vi "InitArm.vi"   [LabVIEW 2020]
uses:
  <vilib>/Rock Robotics/WPI/ThirdParty/Phoenix-LabVIEW/Motor Controller/Controls/CTRE_Phoenix_MotorControl_TalonFXInvertType.ctl
  <vilib>/Rock Robotics/WPI/ThirdParty/Phoenix-LabVIEW/Motor Controller/Controls/CTRE_Phoenix_MotorControl_NeutralMode.ctl
  <vilib>/Rock Robotics/WPI/ThirdParty/Phoenix-LabVIEW/Motor Controller/Controls/CTRE_Phoenix_MotorControl_FeedbackDevice_TalonFX.ctl
  <vilib>/Rock Robotics/WPI/ThirdParty/Phoenix-LabVIEW/Motor Controller/Controls/CTRE_Phoenix_MotorControl_SupplyCurrentLimitConfiguration.ctl
  <vilib>/Rock Robotics/WPI/ThirdParty/Phoenix-LabVIEW/Motor Controller/Controls/CTRE_Phoenix_MotorControl_StatusFrameEnhanced.ctl
  <vilib>/robotics/Kinematics/DH Kinematic Parameters.ctl
  <vilib>/robotics/Kinematics/Link/Joint Type.ctl
  <vilib>/robotics/Kinematics/DH Dynamic Parameters.ctl
  <vilib>/Analysis/Matrix/Datatypes/RealMatrix.ctl
  <vilib>/robotics/Kinematics/RotateX.vi
  <vilib>/robotics/Kinematics/RotateY.vi
  <vilib>/robotics/Kinematics/RotateZ.vi
  <vilib>/Analysis/baseanly.llb/A x B.vi
  <vilib>/Analysis/baseanly.llb/Real A x B.vi
  GlobalArm.vi
  <vilib>/robotics/Kinematics/Analytical/Initialize Generic Serial Arm.vi
  <vilib>/robotics/Kinematics/Robot/NI_Robotics_Serial Robot Arm.lvclass
  <vilib>/robotics/Kinematics/Link/NI_Robotics_Link.lvclass
  <vilib>/robotics/Kinematics/NI_Kinematics.lvlib
  <vilib>/Analysis/Matrix/NI_Matrix.lvlib
  <vilib>/robotics/Kinematics/Analytical/NI_Robotics_AnalyticKinematics.lvlib
types:
  T1 = typedef "CTRE_Phoenix_MotorControl_SupplyCurrentLimitConfiguration.ctl" = cluster{"Enable?":bool, "Current Limit":dbl, "Threshold Current":dbl, "Threshold Time":dbl}
  T2 = typedef "CTRE_Phoenix_MotorControl_NeutralMode.ctl" = enum8{"EEPROMSetting", "Override to Coast", "Override to Brake"}
  T3 = typedef "CTRE_Phoenix_MotorControl_TalonFXInvertType.ctl" = enum16{"Counter-Clockwise", "Clockwise"}
  T4 = typedef "DH Kinematic Parameters.ctl" = cluster{"twist angle":dbl, "length":dbl, "rotation angle":dbl, "offset distance":dbl, "joint type":T5, "joint coordinate offset":dbl}
  T5 = typedef "NI_Robotics_Link.lvclass/Joint Type.ctl" = enum16{"Revolute", "Prismatic"}
  T6 = typedef "CTRE_Phoenix_MotorControl_StatusFrameEnhanced.ctl" = u16
  T7 = typedef "CTRE_Phoenix_MotorControl_FeedbackDevice_TalonFX.ctl" = i8
  T8 = typedef "WPI_MotorControlDeviceRef.ctl" = cluster{"DeviceStatus":errorcluster, "Type":T9, "PWM":cluster{"PWM Channel":T10, "DeadBand":T11}, "CAN":cluster{"Device Number":u8, "SetOutput VI Ref":variant, "GetOutput VI Ref":variant, "Enable VI Ref":variant, "Disable VI Ref":variant, "Data":variant}, "Invert":bool, "DIO PWM":cluster{"PWM \"Enable\" Channel":T10, "DIOChannel":T12, "PWM Rate":dbl}}
  T9 = typedef "WPI_MotorControlType.ctl" = enum16{"PWM", "CAN", "DIO PWM"}
  T10 = typedef "FPGA_DIOPWMChannel.ctl" = enum8{"PWM 0", "PWM 1", "PWM 2", "PWM 3", "PWM 4", "PWM 5", "PWM 6", "PWM 7", "PWM 8", "PWM 9", "PWM MXP 0", "PWM MXP 1", "PWM MXP 2", "PWM MXP 3", "PWM MXP 4", "PWM MXP 5", "PWM MXP 6", "PWM MXP 7", "PWM MXP 8", "PWM MXP 9", "Invalid"}
  T11 = typedef "WPI_PWMDeadband.ctl" = cluster{"Name":string, "maxPositivePwm":i32, "minPositivePwm":i32, "centerPwm":i32, "maxNegativePwm":i32, "minNegativePwm":i32, "angularRange":u16}
  T12 = typedef "FPGA_DIOChannel.ctl" = enum8{"DIO 0", "DIO 1", "DIO 2", "DIO 3", "DIO 4", "DIO 5", "DIO 6", "DIO 7", "DIO 8", "DIO 9", "DIO MXP 0", "DIO MXP 1", "DIO MXP 2", "DIO MXP 3", "DIO MXP 4", "DIO MXP 5", "DIO MXP 6", "DIO MXP 7", "DIO MXP 8", "DIO MXP 9", "DIO MXP 10", "DIO MXP 11", "DIO MXP 12", "DIO MXP 13", "DIO MXP 14", "DIO MXP 15", "SPI Port CS1", "SPI Port CS2", "SPI Port CS3", "SPI Port MISO", "SPI Port MOSI", "Invalid"}
  T13 = typedef "DH Dynamic Parameters.ctl" = cluster{"mass":dbl, "gear ratio":dbl, "motor inertia":dbl, "center of gravity":dbl[], "viscous friction":dbl, "positive coulomb friction":dbl, "negative coulomb friction":dbl, "inertia matrix":T14}
  T14 = typedef "NI_Matrix.lvlib/RealMatrix.ctl" = dbl[][]
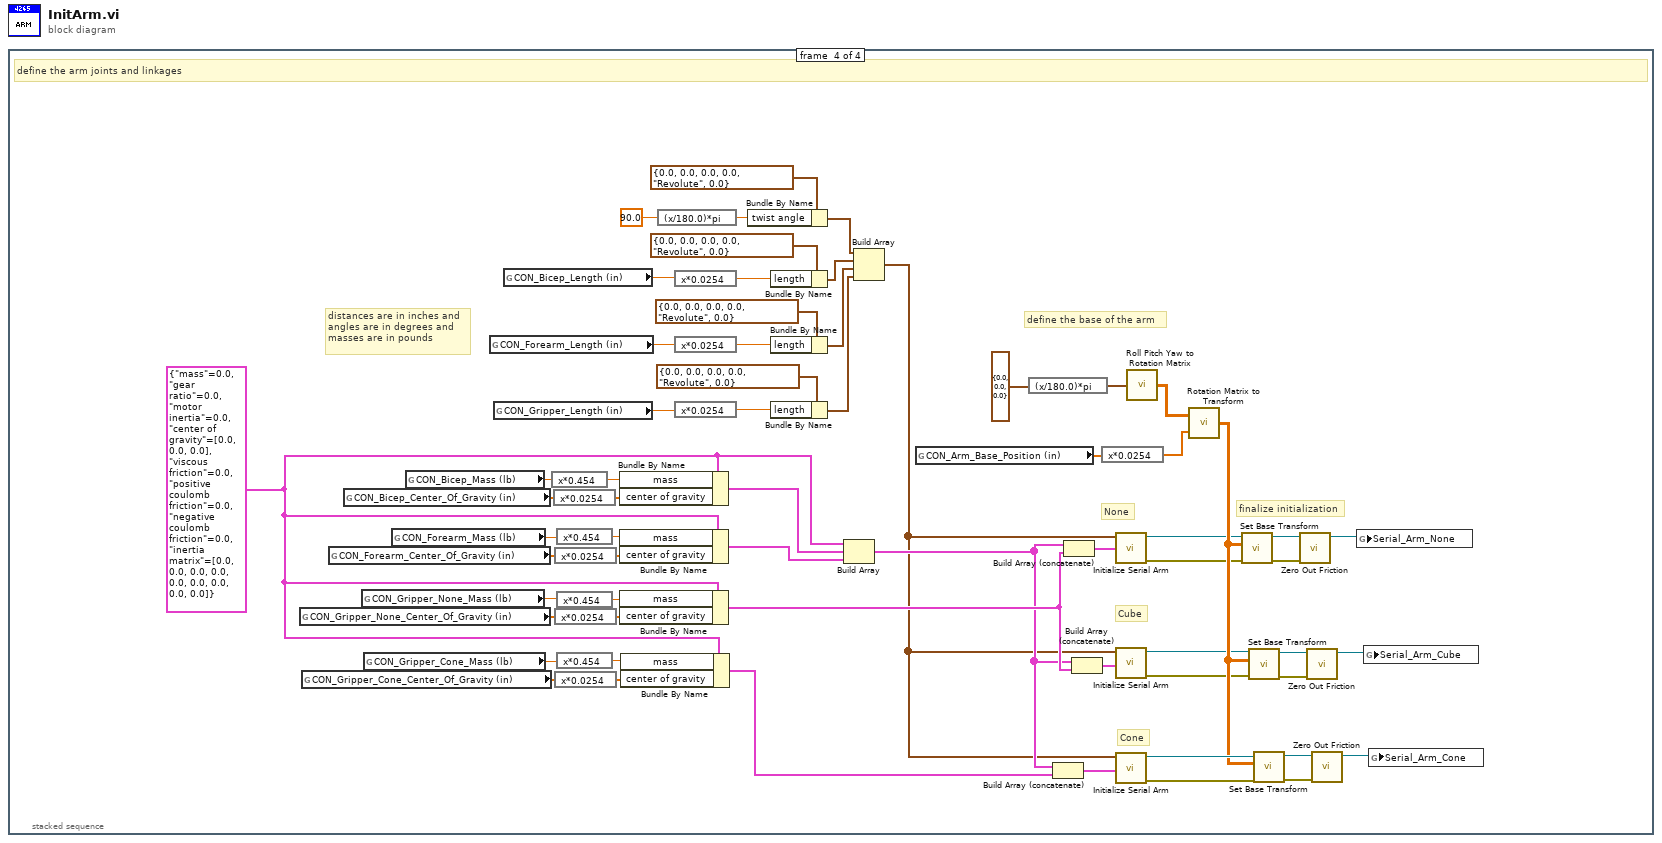
[diagram p0: block diagram]
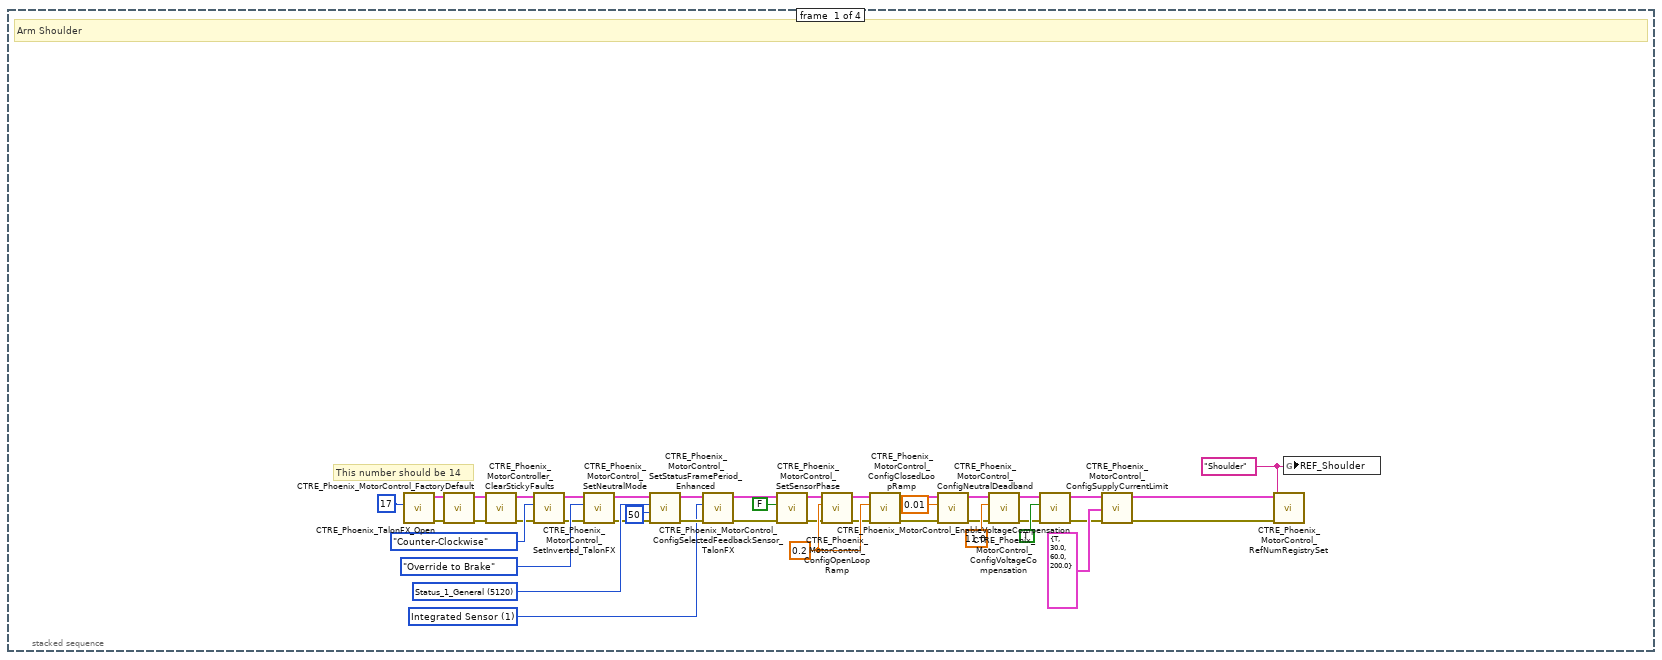
[diagram p2: hidden frame]
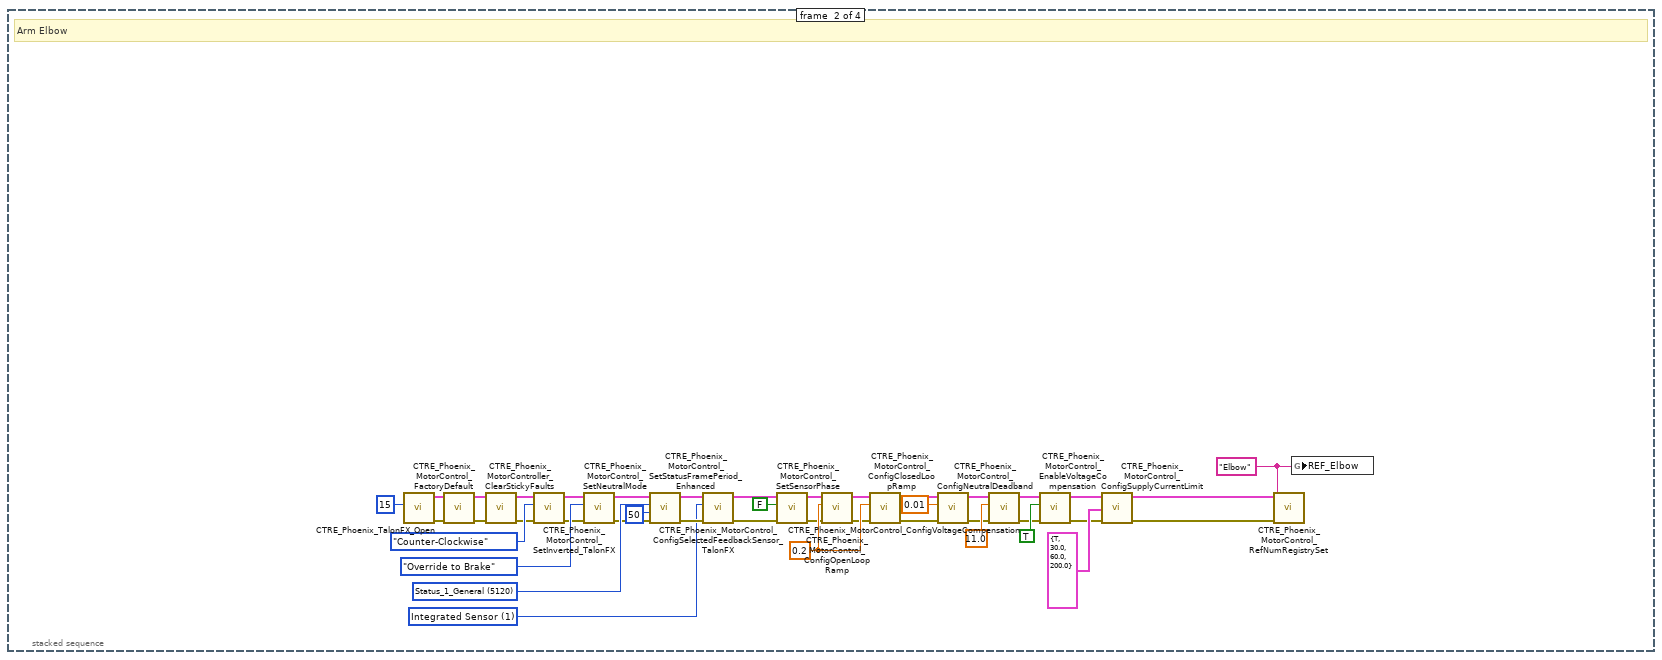
[diagram p3: hidden frame]
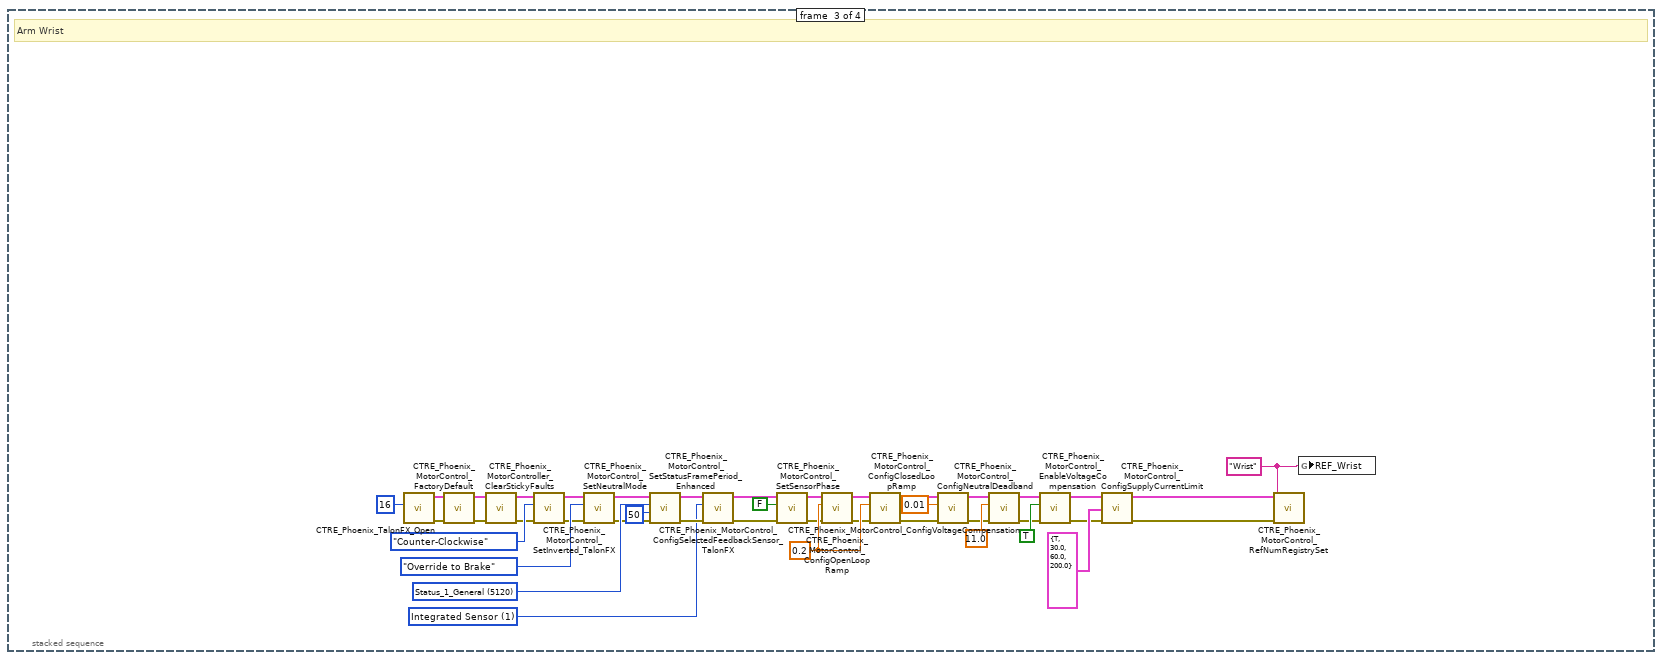
[diagram p4: hidden frame]
diagram:
  n1 = stacked-sequence {
    frame #0 {
      w23 = T6 5120 items=["Status_1_General"=5120, "Status_2_Feedback0"=5184, "Status_3_Quadrature"=5248, "Status_4_AinTempVbat"=5312, "Status_6_Misc"=5440, "Status_7_CommStatus"=5504, "Status_8_PulseWidth"=5568, "Status_9_MotProfBuffer"=5632, "Status_10_MotionMagic"=5696, "Status_11_UartGadgeteer"=5760, "Status_12_Feedback1"=5824, "Status_13_Base_PIDF0"=5888, "Status_14_Turn_PIDF1"=5952, "Status_15_FirmwareApiStatus"=6016, "Status_Brushless_Current"=4672] ("Status Frame")
      w24 = "Shoulder" ("refnum name")
      w28 = 0.2 ("secondsFromNeutralToFull")
      w1 = T7 1 items=["Integrated Sensor"=1, "Sensor Sum (S0 + S1)"=9, "Sensor Difference (D0 - D1)"=10, "Remote Source 0"=11, "Remote Source 1"=12, "None"=14, "Software Emulated"=15] ("Talon FX Feedback Device")
      # "This number should be 14"
      # "Arm Shoulder"
      n2 = call <vilib>:"CTRE_Phoenix_TalonFX_Open.vi"("Device Number"=u8 17) -> ("error out"=w16:errorcluster, "PhoenixMotorControlDevRef"=w33:T8)  [unwired: 9 in]
      n3 = call <vilib>:"CTRE_Phoenix_MotorControl_FactoryDefault.vi"("error in"=w16, "PhoenixMotorControlDevRef"=w33) -> ("error out"=w17:errorcluster, "PhoenixMotorControlDevRef"=w34:T8)  [unwired: 8 in]
      n4 = call <vilib>:"CTRE_Phoenix_MotorController_ClearStickyFaults.vi"("error in"=w17, "PhoenixMotorControlDevRef"=w34) -> ("error out"=w18:errorcluster, "PhoenixMotorControlDevRef"=w35:T8)  [unwired: 8 in]
      n5 = call <vilib>:"CTRE_Phoenix_MotorControl_SetInverted_TalonFX.vi"("error in (no error)"=w18, "Invert Type"=CTRE_Phoenix_MotorControl_TalonFXInvertType."Counter-Clockwise", "PhoenixMotorControlDevRef"=w35) -> ("error out"=w19:errorcluster, "PhoenixMotorControlDevRef"=w36:T8)  [unwired: 7 in]
      n6 = call <vilib>:"CTRE_Phoenix_MotorControl_SetNeutralMode.vi"("error in (no error)"=w19, "Motor Control Neutral Mode"=CTRE_Phoenix_MotorControl_NeutralMode."Override to Brake", "PhoenixMotorControlDevRef"=w36) -> ("error out"=w20:errorcluster, "PhoenixMotorControlDevRef"=w41:T8)  [unwired: 7 in]
      n7 = call <vilib>:"CTRE_Phoenix_MotorControl_SetStatusFramePeriod_Enhanced.vi"("error in (no error)"=w20, "periodMs"=50, "Status Frame"=w23, "PhoenixMotorControlDevRef"=w41) -> ("error out"=w21:errorcluster, "PhoenixMotorControlDevRef"=w22:T8)  [unwired: 6 in]
      n8 = call <vilib>:"CTRE_Phoenix_MotorControl_ConfigSelectedFeedbackSensor_TalonFX.vi"("error in (no error)"=w21, "Talon FX Feedback Device"=w1, "PhoenixMotorControlDevRef"=w22) -> ("error out"=w9:errorcluster, "PhoenixMotorControlDevRef"=w11:T8)  [unwired: 7 in]
      n9 = call <vilib>:"CTRE_Phoenix_MotorControl_SetSensorPhase.vi"("error in (no error)"=w9, "PhaseSensor"=FALSE, "PhoenixMotorControlDevRef"=w11) -> ("error out"=w8:errorcluster, "PhoenixMotorControlDevRef"=w10:T8)  [unwired: 7 in]
      n10 = call <vilib>:"CTRE_Phoenix_MotorControl_ConfigOpenLoopRamp.vi"("error in (no error)"=w8, "secondsFromNeutralToFull"=w28, "PhoenixMotorControlDevRef"=w10) -> ("error out"=w15:errorcluster, "PhoenixMotorControlDevRef"=w37:T8)  [unwired: 7 in]
      n11 = call <vilib>:"CTRE_Phoenix_MotorControl_ConfigClosedLoopRamp.vi"("error in (no error)"=w15, "secondsFromNeutralToFull"=w28, "PhoenixMotorControlDevRef"=w37) -> ("error out"=w5:errorcluster, "PhoenixMotorControlDevRef"=w6:T8)  [unwired: 7 in]
      n12 = call <vilib>:"CTRE_Phoenix_MotorControl_ConfigNeutralDeadband.vi"("error in (no error)"=w5, "Percent Deadband"=0.01, "PhoenixMotorControlDevRef"=w6) -> ("error out"=w4:errorcluster, "PhoenixMotorControlDevRef"=w3:T8)  [unwired: 7 in]
      n13 = call <vilib>:"CTRE_Phoenix_MotorControl_ConfigVoltageCompensation.vi"("error in (no error)"=w4, "Saturation Voltage"=11.0, "PhoenixMotorControlDevRef"=w3) -> ("error out"=w14:errorcluster, "PhoenixMotorControlDevRef"=w38:T8)  [unwired: 7 in]
      n14 = call <vilib>:"CTRE_Phoenix_MotorControl_EnableVoltageCompensation.vi"("error in (no error)"=w14, "Enable Voltage Compensation?"=TRUE, "PhoenixMotorControlDevRef"=w38) -> ("error out"=w13:errorcluster, "PhoenixMotorControlDevRef"=w39:T8)  [unwired: 7 in]
      n15 = call <vilib>:"CTRE_Phoenix_MotorControl_ConfigSupplyCurrentLimit.vi"("error in (no error)"=w13, "Supply Current Limit Configuration"=T1 {"Enable?"=TRUE, "Current Limit"=30.0, "Threshold Current"=60.0, "Threshold Time"=200.0}, "PhoenixMotorControlDevRef"=w39) -> ("error out"=w12:errorcluster, "PhoenixMotorControlDevRef"=w40:T8)  [unwired: 7 in]
      n16 = call <vilib>:"CTRE_Phoenix_MotorControl_RefNumRegistrySet.vi"("error in (no error)"=w12, "refnum name"=w24, "PhoenixMotorControlDevRef"=w40) -> ()  [unwired: 7 in, 2 out]
      n17 = global write "GlobalArm.vi" "REF_Shoulder"(w24) -> ()
    }
    frame #1 {
      w64 = T6 5120 items=["Status_1_General"=5120, "Status_2_Feedback0"=5184, "Status_3_Quadrature"=5248, "Status_4_AinTempVbat"=5312, "Status_6_Misc"=5440, "Status_7_CommStatus"=5504, "Status_8_PulseWidth"=5568, "Status_9_MotProfBuffer"=5632, "Status_10_MotionMagic"=5696, "Status_11_UartGadgeteer"=5760, "Status_12_Feedback1"=5824, "Status_13_Base_PIDF0"=5888, "Status_14_Turn_PIDF1"=5952, "Status_15_FirmwareApiStatus"=6016, "Status_Brushless_Current"=4672] ("Status Frame")
      w65 = "Elbow" ("refnum name")
      w69 = 0.2 ("secondsFromNeutralToFull")
      w42 = T7 1 items=["Integrated Sensor"=1, "Sensor Sum (S0 + S1)"=9, "Sensor Difference (D0 - D1)"=10, "Remote Source 0"=11, "Remote Source 1"=12, "None"=14, "Software Emulated"=15] ("Talon FX Feedback Device")
      # "Arm Elbow"
      n18 = call <vilib>:"CTRE_Phoenix_TalonFX_Open.vi"("Device Number"=u8 15) -> ("error out"=w57:errorcluster, "PhoenixMotorControlDevRef"=w74:T8)  [unwired: 9 in]
      n19 = call <vilib>:"CTRE_Phoenix_MotorControl_FactoryDefault.vi"("error in"=w57, "PhoenixMotorControlDevRef"=w74) -> ("error out"=w58:errorcluster, "PhoenixMotorControlDevRef"=w75:T8)  [unwired: 8 in]
      n20 = call <vilib>:"CTRE_Phoenix_MotorController_ClearStickyFaults.vi"("error in"=w58, "PhoenixMotorControlDevRef"=w75) -> ("error out"=w59:errorcluster, "PhoenixMotorControlDevRef"=w76:T8)  [unwired: 8 in]
      n21 = call <vilib>:"CTRE_Phoenix_MotorControl_SetInverted_TalonFX.vi"("error in (no error)"=w59, "Invert Type"=CTRE_Phoenix_MotorControl_TalonFXInvertType."Counter-Clockwise", "PhoenixMotorControlDevRef"=w76) -> ("error out"=w60:errorcluster, "PhoenixMotorControlDevRef"=w77:T8)  [unwired: 7 in]
      n22 = call <vilib>:"CTRE_Phoenix_MotorControl_SetNeutralMode.vi"("error in (no error)"=w60, "Motor Control Neutral Mode"=CTRE_Phoenix_MotorControl_NeutralMode."Override to Brake", "PhoenixMotorControlDevRef"=w77) -> ("error out"=w61:errorcluster, "PhoenixMotorControlDevRef"=w82:T8)  [unwired: 7 in]
      n23 = call <vilib>:"CTRE_Phoenix_MotorControl_SetStatusFramePeriod_Enhanced.vi"("error in (no error)"=w61, "periodMs"=50, "Status Frame"=w64, "PhoenixMotorControlDevRef"=w82) -> ("error out"=w62:errorcluster, "PhoenixMotorControlDevRef"=w63:T8)  [unwired: 6 in]
      n24 = call <vilib>:"CTRE_Phoenix_MotorControl_ConfigSelectedFeedbackSensor_TalonFX.vi"("error in (no error)"=w62, "Talon FX Feedback Device"=w42, "PhoenixMotorControlDevRef"=w63) -> ("error out"=w50:errorcluster, "PhoenixMotorControlDevRef"=w52:T8)  [unwired: 7 in]
      n25 = call <vilib>:"CTRE_Phoenix_MotorControl_SetSensorPhase.vi"("error in (no error)"=w50, "PhaseSensor"=FALSE, "PhoenixMotorControlDevRef"=w52) -> ("error out"=w49:errorcluster, "PhoenixMotorControlDevRef"=w51:T8)  [unwired: 7 in]
      n26 = call <vilib>:"CTRE_Phoenix_MotorControl_ConfigOpenLoopRamp.vi"("error in (no error)"=w49, "secondsFromNeutralToFull"=w69, "PhoenixMotorControlDevRef"=w51) -> ("error out"=w56:errorcluster, "PhoenixMotorControlDevRef"=w78:T8)  [unwired: 7 in]
      n27 = call <vilib>:"CTRE_Phoenix_MotorControl_ConfigClosedLoopRamp.vi"("error in (no error)"=w56, "secondsFromNeutralToFull"=w69, "PhoenixMotorControlDevRef"=w78) -> ("error out"=w46:errorcluster, "PhoenixMotorControlDevRef"=w47:T8)  [unwired: 7 in]
      n28 = call <vilib>:"CTRE_Phoenix_MotorControl_ConfigNeutralDeadband.vi"("error in (no error)"=w46, "Percent Deadband"=0.01, "PhoenixMotorControlDevRef"=w47) -> ("error out"=w45:errorcluster, "PhoenixMotorControlDevRef"=w44:T8)  [unwired: 7 in]
      n29 = call <vilib>:"CTRE_Phoenix_MotorControl_ConfigVoltageCompensation.vi"("error in (no error)"=w45, "Saturation Voltage"=11.0, "PhoenixMotorControlDevRef"=w44) -> ("error out"=w55:errorcluster, "PhoenixMotorControlDevRef"=w79:T8)  [unwired: 7 in]
      n30 = call <vilib>:"CTRE_Phoenix_MotorControl_EnableVoltageCompensation.vi"("error in (no error)"=w55, "Enable Voltage Compensation?"=TRUE, "PhoenixMotorControlDevRef"=w79) -> ("error out"=w54:errorcluster, "PhoenixMotorControlDevRef"=w80:T8)  [unwired: 7 in]
      n31 = call <vilib>:"CTRE_Phoenix_MotorControl_ConfigSupplyCurrentLimit.vi"("error in (no error)"=w54, "Supply Current Limit Configuration"=T1 {"Enable?"=TRUE, "Current Limit"=30.0, "Threshold Current"=60.0, "Threshold Time"=200.0}, "PhoenixMotorControlDevRef"=w80) -> ("error out"=w53:errorcluster, "PhoenixMotorControlDevRef"=w81:T8)  [unwired: 7 in]
      n32 = call <vilib>:"CTRE_Phoenix_MotorControl_RefNumRegistrySet.vi"("error in (no error)"=w53, "refnum name"=w65, "PhoenixMotorControlDevRef"=w81) -> ()  [unwired: 7 in, 2 out]
      n33 = global write "GlobalArm.vi" "REF_Elbow"(w65) -> ()
    }
    frame #2 {
      w106 = T6 5120 items=["Status_1_General"=5120, "Status_2_Feedback0"=5184, "Status_3_Quadrature"=5248, "Status_4_AinTempVbat"=5312, "Status_6_Misc"=5440, "Status_7_CommStatus"=5504, "Status_8_PulseWidth"=5568, "Status_9_MotProfBuffer"=5632, "Status_10_MotionMagic"=5696, "Status_11_UartGadgeteer"=5760, "Status_12_Feedback1"=5824, "Status_13_Base_PIDF0"=5888, "Status_14_Turn_PIDF1"=5952, "Status_15_FirmwareApiStatus"=6016, "Status_Brushless_Current"=4672] ("Status Frame")
      w110 = 0.2 ("secondsFromNeutralToFull")
      w83 = T7 1 items=["Integrated Sensor"=1, "Sensor Sum (S0 + S1)"=9, "Sensor Difference (D0 - D1)"=10, "Remote Source 0"=11, "Remote Source 1"=12, "None"=14, "Software Emulated"=15] ("Talon FX Feedback Device")
      w84 = "Wrist" ("refnum name")
      # "Arm Wrist"
      n34 = call <vilib>:"CTRE_Phoenix_TalonFX_Open.vi"("Device Number"=u8 16) -> ("error out"=w99:errorcluster, "PhoenixMotorControlDevRef"=w115:T8)  [unwired: 9 in]
      n35 = call <vilib>:"CTRE_Phoenix_MotorControl_FactoryDefault.vi"("error in"=w99, "PhoenixMotorControlDevRef"=w115) -> ("error out"=w100:errorcluster, "PhoenixMotorControlDevRef"=w116:T8)  [unwired: 8 in]
      n36 = call <vilib>:"CTRE_Phoenix_MotorController_ClearStickyFaults.vi"("error in"=w100, "PhoenixMotorControlDevRef"=w116) -> ("error out"=w101:errorcluster, "PhoenixMotorControlDevRef"=w117:T8)  [unwired: 8 in]
      n37 = call <vilib>:"CTRE_Phoenix_MotorControl_SetInverted_TalonFX.vi"("error in (no error)"=w101, "Invert Type"=CTRE_Phoenix_MotorControl_TalonFXInvertType."Counter-Clockwise", "PhoenixMotorControlDevRef"=w117) -> ("error out"=w102:errorcluster, "PhoenixMotorControlDevRef"=w118:T8)  [unwired: 7 in]
      n38 = call <vilib>:"CTRE_Phoenix_MotorControl_SetNeutralMode.vi"("error in (no error)"=w102, "Motor Control Neutral Mode"=CTRE_Phoenix_MotorControl_NeutralMode."Override to Brake", "PhoenixMotorControlDevRef"=w118) -> ("error out"=w103:errorcluster, "PhoenixMotorControlDevRef"=w123:T8)  [unwired: 7 in]
      n39 = call <vilib>:"CTRE_Phoenix_MotorControl_SetStatusFramePeriod_Enhanced.vi"("error in (no error)"=w103, "periodMs"=50, "Status Frame"=w106, "PhoenixMotorControlDevRef"=w123) -> ("error out"=w104:errorcluster, "PhoenixMotorControlDevRef"=w105:T8)  [unwired: 6 in]
      n40 = call <vilib>:"CTRE_Phoenix_MotorControl_ConfigSelectedFeedbackSensor_TalonFX.vi"("error in (no error)"=w104, "Talon FX Feedback Device"=w83, "PhoenixMotorControlDevRef"=w105) -> ("error out"=w92:errorcluster, "PhoenixMotorControlDevRef"=w94:T8)  [unwired: 7 in]
      n41 = call <vilib>:"CTRE_Phoenix_MotorControl_SetSensorPhase.vi"("error in (no error)"=w92, "PhaseSensor"=FALSE, "PhoenixMotorControlDevRef"=w94) -> ("error out"=w91:errorcluster, "PhoenixMotorControlDevRef"=w93:T8)  [unwired: 7 in]
      n42 = call <vilib>:"CTRE_Phoenix_MotorControl_ConfigOpenLoopRamp.vi"("error in (no error)"=w91, "secondsFromNeutralToFull"=w110, "PhoenixMotorControlDevRef"=w93) -> ("error out"=w98:errorcluster, "PhoenixMotorControlDevRef"=w119:T8)  [unwired: 7 in]
      n43 = call <vilib>:"CTRE_Phoenix_MotorControl_ConfigClosedLoopRamp.vi"("error in (no error)"=w98, "secondsFromNeutralToFull"=w110, "PhoenixMotorControlDevRef"=w119) -> ("error out"=w88:errorcluster, "PhoenixMotorControlDevRef"=w89:T8)  [unwired: 7 in]
      n44 = call <vilib>:"CTRE_Phoenix_MotorControl_ConfigNeutralDeadband.vi"("error in (no error)"=w88, "Percent Deadband"=0.01, "PhoenixMotorControlDevRef"=w89) -> ("error out"=w87:errorcluster, "PhoenixMotorControlDevRef"=w86:T8)  [unwired: 7 in]
      n45 = call <vilib>:"CTRE_Phoenix_MotorControl_ConfigVoltageCompensation.vi"("error in (no error)"=w87, "Saturation Voltage"=11.0, "PhoenixMotorControlDevRef"=w86) -> ("error out"=w97:errorcluster, "PhoenixMotorControlDevRef"=w120:T8)  [unwired: 7 in]
      n46 = call <vilib>:"CTRE_Phoenix_MotorControl_EnableVoltageCompensation.vi"("error in (no error)"=w97, "Enable Voltage Compensation?"=TRUE, "PhoenixMotorControlDevRef"=w120) -> ("error out"=w96:errorcluster, "PhoenixMotorControlDevRef"=w121:T8)  [unwired: 7 in]
      n47 = call <vilib>:"CTRE_Phoenix_MotorControl_ConfigSupplyCurrentLimit.vi"("error in (no error)"=w96, "Supply Current Limit Configuration"=T1 {"Enable?"=TRUE, "Current Limit"=30.0, "Threshold Current"=60.0, "Threshold Time"=200.0}, "PhoenixMotorControlDevRef"=w121) -> ("error out"=w95:errorcluster, "PhoenixMotorControlDevRef"=w122:T8)  [unwired: 7 in]
      n48 = call <vilib>:"CTRE_Phoenix_MotorControl_RefNumRegistrySet.vi"("error in (no error)"=w95, "refnum name"=w84, "PhoenixMotorControlDevRef"=w122) -> ()  [unwired: 7 in, 2 out]
      n49 = global write "GlobalArm.vi" "REF_Wrist"(w84) -> ()
    }
    frame #3 {
      w124 = T13 {"mass"=0.0, "gear ratio"=0.0, "motor inertia"=0.0, "center of gravity"=[0.0, 0.0, 0.0], "viscous friction"=0.0, "positive coulomb friction"=0.0, "negative coulomb friction"=0.0, "inertia matrix"=[[0.0, 0.0, 0.0], [0.0, 0.0, 0.0], [0.0, 0.0, 0.0]]} ("dynamic parameters")
      # "Cube"
      # "None"
      # "Cone"
      # "define the base of the arm"
      # "distances are in inches and\nangles are in degrees and\nmasses are in pounds"
      # "finalize initialization"
      # "define the arm joints and linkages"
      n50 = global read "GlobalArm.vi" "CON_Gripper_None_Center_Of_Gravity (in)"() -> (w166:dbl[])
      n51 = global read "GlobalArm.vi" "CON_Gripper_Cone_Center_Of_Gravity (in)"() -> (w168:dbl[])
      n52 = global read "GlobalArm.vi" "CON_Forearm_Center_Of_Gravity (in)"() -> (w162:dbl[])
      n53 = global read "GlobalArm.vi" "CON_Bicep_Center_Of_Gravity (in)"() -> (w165:dbl[])
      n54 = global read "GlobalArm.vi" "CON_Gripper_None_Mass (lb)"() -> (w174:dbl)
      n55 = global read "GlobalArm.vi" "CON_Gripper_Cone_Mass (lb)"() -> (w176:dbl)
      n56 = global read "GlobalArm.vi" "CON_Forearm_Mass (lb)"() -> (w172:dbl)
      n57 = global read "GlobalArm.vi" "CON_Bicep_Mass (lb)"() -> (w170:dbl)
      n58 = global read "GlobalArm.vi" "CON_Forearm_Length (in)"() -> (w155:dbl)
      n59 = global read "GlobalArm.vi" "CON_Gripper_Length (in)"() -> (w153:dbl)
      n60 = global read "GlobalArm.vi" "CON_Bicep_Length (in)"() -> (w154:dbl)
      n61 = expression code="x*0.454" ("degrees to radians")(w170) -> (w171:dbl)
      n62 = expression code="x*0.0254" ("degrees to radians")(w165) -> (w164:dbl[])
      n63 = expression code="x*0.0254" ("degrees to radians")(w162) -> (w163:dbl[])
      n64 = expression code="x*0.0254" ("degrees to radians")(w166) -> (w167:dbl[])
      n65 = expression code="x*0.0254" ("degrees to radians")(w168) -> (w169:dbl[])
      n66 = expression code="x*0.454" ("degrees to radians")(w172) -> (w173:dbl)
      n67 = expression code="x*0.454" ("degrees to radians")(w174) -> (w175:dbl)
      n68 = expression code="x*0.454" ("degrees to radians")(w176) -> (w177:dbl)
      n69 = Bundle By Name(cluster=w124, "mass"=w171, "center of gravity"=w164) -> (w156:T13)
      n70 = Bundle By Name(cluster=w124, "mass"=w173, "center of gravity"=w163) -> (w157:T13)
      n71 = Bundle By Name(cluster=w124, "mass"=w175, "center of gravity"=w167) -> (w159:T13)
      n72 = Bundle By Name(cluster=w124, "mass"=w177, "center of gravity"=w169) -> (w160:T13)
      n73 = expression code="(x/180.0)*pi" ("degrees to radians")(90.0 ("twist angle")) -> (w136:dbl)
      n74 = expression code="x*0.0254" ("degrees to radians")(w154) -> (w131:dbl)
      n75 = expression code="x*0.0254" ("degrees to radians")(w155) -> (w149:dbl)
      n76 = expression code="x*0.0254" ("degrees to radians")(w153) -> (w150:dbl)
      n77 = Bundle By Name(cluster=T4 {"twist angle"=0.0, "length"=0.0, "rotation angle"=0.0, "offset distance"=0.0, "joint type"=enum."Revolute", "joint coordinate offset"=0.0} ("Link Parameters"), "twist angle"=w136) -> (w137:T4)
      n78 = Bundle By Name(cluster=T4 {"twist angle"=0.0, "length"=0.0, "rotation angle"=0.0, "offset distance"=0.0, "joint type"=enum."Revolute", "joint coordinate offset"=0.0} ("Link Parameters"), "length"=w131) -> (w132:T4)
      n79 = Bundle By Name(cluster=T4 {"twist angle"=0.0, "length"=0.0, "rotation angle"=0.0, "offset distance"=0.0, "joint type"=enum."Revolute", "joint coordinate offset"=0.0} ("Link Parameters"), "length"=w149) -> (w152:T4)
      n80 = Bundle By Name(cluster=T4 {"twist angle"=0.0, "length"=0.0, "rotation angle"=0.0, "offset distance"=0.0, "joint type"=enum."Revolute", "joint coordinate offset"=0.0} ("Link Parameters"), "length"=w150) -> (w151:T4)
      n81 = Build Array(w124, w156, w157) -> (w158:T13[])
      n82 = Build Array(w137, w132, w152, w151) -> (w142:T4[])
      n83 = global read "GlobalArm.vi" "CON_Arm_Base_Position (in)"() -> (w161:dbl[])
      n84 = expression code="(x/180.0)*pi" ("degrees to radians")(cluster{"roll":dbl, "pitch":dbl, "yaw":dbl} {"roll"=0.0, "pitch"=0.0, "yaw"=0.0} ("angles")) -> (w134:cluster{"roll":dbl, "pitch":dbl, "yaw":dbl})
      n85 = Build Array (concatenate)(w158, w160) -> (w141:T13[])
      n86 = Build Array (concatenate)(w158, w159) -> (w148:T13[])
      n87 = Build Array (concatenate)(w158, w159) -> (w140:T13[])
      n88 = expression code="x*0.0254" ("degrees to radians")(w161) -> (w135:dbl[])
      n89 = call-poly <vilib>:"Initialize Serial Arm.vi"("dynamic parameters"=w148, "kinematic parameters"=w142) -> ("error out"=w138:errorcluster, "serial arm out"=w139:refnum<class "NI_Robotics_Serial Robot Arm.lvclass">)  [unwired: 8 in]
      n90 = call-poly <vilib>:"Initialize Serial Arm.vi"("dynamic parameters"=w140, "kinematic parameters"=w142) -> ("error out"=w144:errorcluster, "serial arm out"=w143:refnum<class "NI_Robotics_Serial Robot Arm.lvclass">)  [unwired: 8 in]
      n91 = call-poly <vilib>:"Initialize Serial Arm.vi"("dynamic parameters"=w141, "kinematic parameters"=w142) -> ("error out"=w147:errorcluster, "serial arm out"=w146:refnum<class "NI_Robotics_Serial Robot Arm.lvclass">)  [unwired: 8 in]
      n92 = call <vilib>:"Roll Pitch Yaw to Rotation Matrix.vi"("angles"=w134) -> ("rotation matrix"=w133:T14)
      n93 = call <vilib>:"Rotation Matrix to Transform.vi"("translation vector"=w135, "rotation matrix"=w133) -> ("transform"=w145:T14)
      n94 = call <vilib>:"Set Base Transform.vi"("error in (no error)"=w138, "base transform"=w145, "serial arm in"=w139) -> ("error out"=w184:errorcluster, "serial arm out"=w183:refnum<class "NI_Robotics_Serial Robot Arm.lvclass">)  [unwired: 7 in]
      n95 = call <vilib>:"Set Base Transform.vi"("error in (no error)"=w144, "base transform"=w145, "serial arm in"=w143) -> ("error out"=w182:errorcluster, "serial arm out"=w181:refnum<class "NI_Robotics_Serial Robot Arm.lvclass">)  [unwired: 7 in]
      n96 = call <vilib>:"Set Base Transform.vi"("error in (no error)"=w147, "base transform"=w145, "serial arm in"=w146) -> ("error out"=w186:errorcluster, "serial arm out"=w185:refnum<class "NI_Robotics_Serial Robot Arm.lvclass">)  [unwired: 7 in]
      n97 = call <vilib>:"Zero Out Friction.vi"("error in (no error)"=w184, "serial arm in"=w183) -> ("serial arm out"=w178:refnum<class "NI_Robotics_Serial Robot Arm.lvclass">)  [unwired: 8 in, 1 out]
      n98 = call <vilib>:"Zero Out Friction.vi"("error in (no error)"=w182, "serial arm in"=w181) -> ("serial arm out"=w179:refnum<class "NI_Robotics_Serial Robot Arm.lvclass">)  [unwired: 8 in, 1 out]
      n99 = call <vilib>:"Zero Out Friction.vi"("error in (no error)"=w186, "serial arm in"=w185) -> ("serial arm out"=w180:refnum<class "NI_Robotics_Serial Robot Arm.lvclass">)  [unwired: 8 in, 1 out]
      n100 = global write "GlobalArm.vi" "Serial_Arm_None"(w178) -> ()
      n101 = global write "GlobalArm.vi" "Serial_Arm_Cube"(w179) -> ()
      n102 = global write "GlobalArm.vi" "Serial_Arm_Cone"(w180) -> ()
    }
  }
